vi "Test Post-filter.vi"(8 "error in (no error)":errorcluster, 11 "Lockin.DAQ in":refnum<class "Instrument.DAQ.lvclass">) -> (0 "error out":errorcluster, 3 "Lockin.DAQ out":refnum<class "Instrument.DAQ.lvclass">)   [LabVIEW 2019, in "Instrument.Lockin.lvlib" / "Instrument.DAQ.lvclass"]
uses:
  Instrument.DAQ.lvclass
  DSP/DSP.lvclass
  Typedefs/AO.Channel.Function--Enum.ctl
  Typedefs/AO.Channel--Cluster--Array.ctl
  Typedefs/REF.Channel--Cluster--Array.ctl
  Typedefs/DAQ.Sampling.Sampling--Cluster.ctl
  Typedefs/AO.Channel--Cluster.ctl
  Typedefs/REF.Channel--Cluster.ctl
  Typedefs/AI.Channel--Cluster.ctl
  Typedefs/AI.Channel--Cluster--Array.ctl
panel:
  out "appended array":waveform(dbl)[](array[waveform])
  out "Waveform Graph":waveform(dbl)[](graph)
  in  "AI Channels":T1 {"References" items=["", "1", "2", "3"]; "Channel" min=1}
  in  "REF Channels":T3 {"Roll-Off" min=1; "TC" min=0.0001 format="%#_3p"; "Phase" format="%.3g"; "Frequency" min=0.0001 max=10000.0 format="%.3g"; "Channel" min=1}
  in  "sampling":T5={"Fs"=204789.0, "#s"=15753} {"Fs" format="%#_13g"}
  in  "stop":bool
  in  "AO Channels":T6=[{"Enable?"=FALSE, "Channel"=0, "Amplitude"=0.0, "Offset"=0.0, "Frequency"=0.1, "Phase"=0.0, "Function"=enum."Sine", "Sweeping?"=FALSE, "Limit AC"=FALSE, "Limit DC?"=FALSE}] {"Phase" format="%.2g"; "Frequency" min=0.0001 max=10000.0 format="%.2g"; "Offset" format="%5.2p"; "Amplitude" min=0.0 max=10.0 format="%5.2p"}
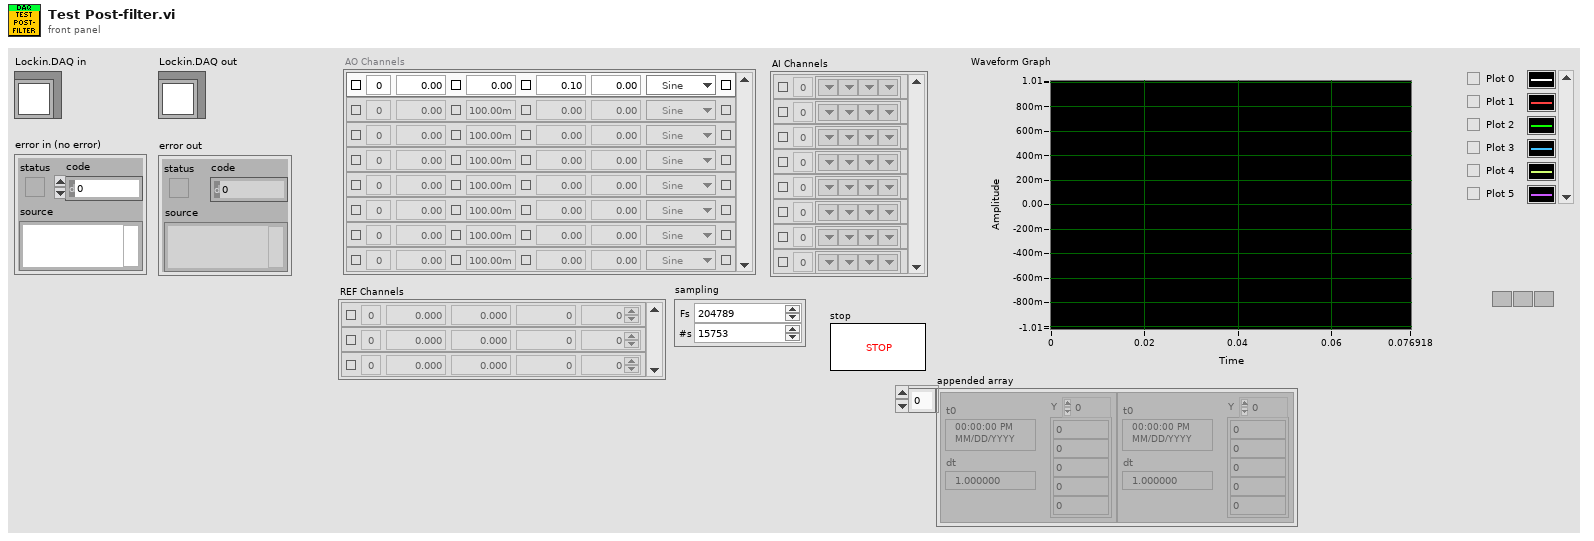
[diagram p1: front panel]
types:
  T1 = typedef "Instrument.Lockin.lvlib/Instrument.DAQ.lvclass/AI.Channel--Cluster--Array.ctl" = T2[]
  T2 = typedef "Instrument.Lockin.lvlib/Instrument.DAQ.lvclass/AI.Channel--Cluster.ctl" = cluster{"Enable?":bool, "Channel":i32, "References":i32[]}
  T3 = typedef "Instrument.Lockin.lvlib/Instrument.DAQ.lvclass/REF.Channel--Cluster--Array.ctl" = T4[]
  T4 = typedef "Instrument.Lockin.lvlib/Instrument.DAQ.lvclass/REF.Channel--Cluster.ctl" = cluster{"Enable?":bool, "Channel":i32, "Frequency":dbl, "Phase":dbl, "TC":dbl, "Roll-Off":i32}
  T5 = typedef "Instrument.Lockin.lvlib/Instrument.DAQ.lvclass/DAQ.Sampling.Sampling--Cluster.ctl" = cluster{"Fs":dbl, "#s":i32}
  T6 = typedef "Instrument.Lockin.lvlib/Instrument.DAQ.lvclass/AO.Channel--Cluster--Array.ctl" = T7[]
  T7 = typedef "Instrument.Lockin.lvlib/Instrument.DAQ.lvclass/AO.Channel--Cluster.ctl" = cluster{"Enable?":bool, "Channel":i32, "Amplitude":dbl, "Offset":dbl, "Frequency":dbl, "Phase":dbl, "Function":T8, "Sweeping?":bool, "Limit AC":bool, "Limit DC?":bool}
  T8 = typedef "Instrument.Lockin.lvlib/Instrument.DAQ.lvclass/AO.Channel.Function--Enum.ctl" = enum16{"Sine", "Triangle", "Square"}
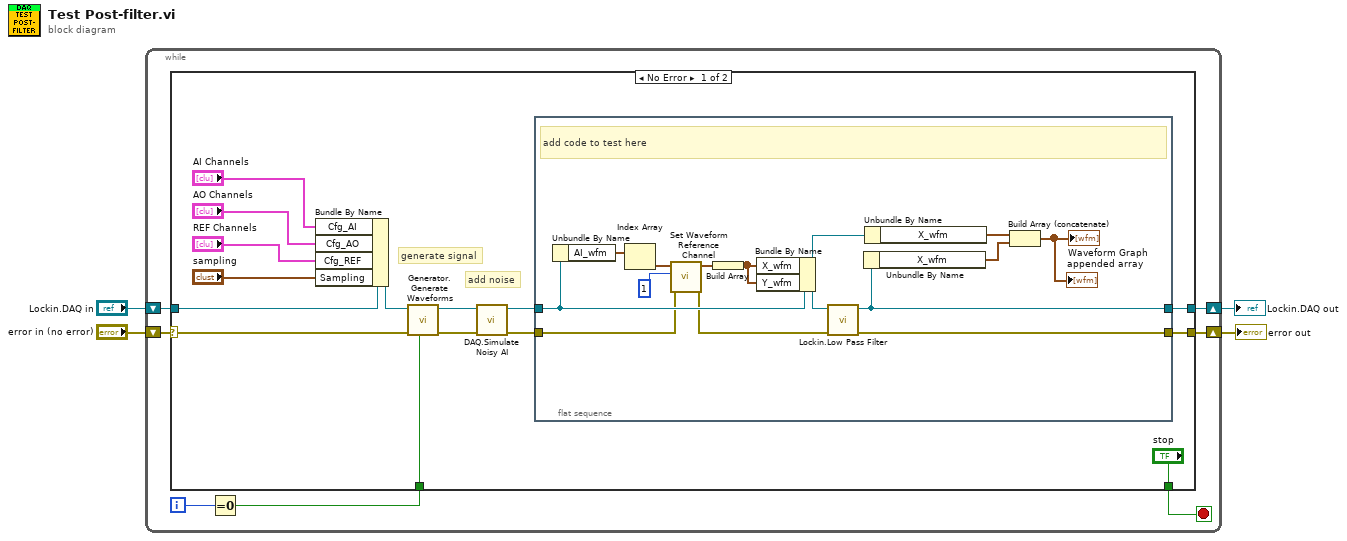
[diagram p0: block diagram]
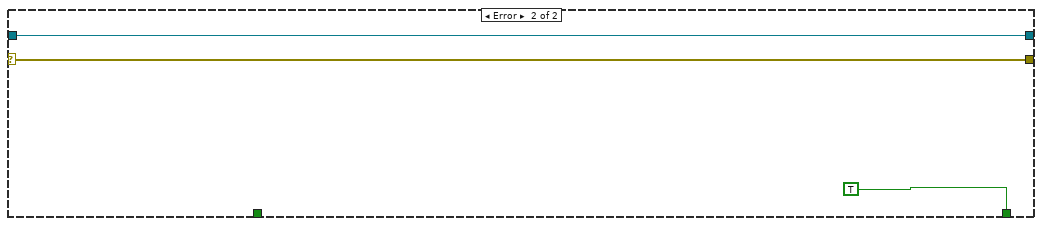
[diagram p2: hidden frame]
diagram:
  n1 = while {
    shift-right: [w10] -> w3
    shift-left: "error in (no error)" -> [w11]
    shift-right: [w8] -> w1
    shift-left: "Lockin.DAQ in" -> [w9]
    i -> [w6]
    stop <- w5 stop-if-true
    n2 = Equal To 0?(x=w6) -> (x = 0?=w7:bool)
    n3 = case shown="No Error" w11 {
      selector: w11 -> [w25 w43]
      tunnel: [w22 w43] -> w10
      tunnel: [w24 w42] -> w8
      tunnel: w9 -> [w15 w42]
      tunnel: w7 -> [w21 _]
      tunnel: ["stop" TRUE ("stop")] -> w5
      frame No Error {
        # "generate signal"
        # "add noise"
        n4 = Bundle By Name(cluster=w15, "Cfg_AI"="AI Channels", "Cfg_AO"="AO Channels", "Cfg_REF"="REF Channels", "Sampling"="sampling") -> (w16:refnum<class "Instrument.DAQ.lvclass">)
        n5 = call "Generator.Generate Waveforms.vi"("Reset Phase?"=w21, "error in (no error)"=w25, "Instrument.DAQ"=w16) -> ("error out"=w26:errorcluster, "Instrument.DAQ"=w12:refnum<class "Instrument.DAQ.lvclass">)  [unwired: 7 in]
        n6 = call "DAQ.Simulate Noisy AI.vi"("error in (no error)"=w26, "Instrument.DAQ in"=w12) -> ("error out"=w23:errorcluster, "Instrument.DAQ out"=w13:refnum<class "Instrument.DAQ.lvclass">)  [unwired: 6 in, 2 out]
        n7 = flat-sequence {
          tunnel: [w35] -> w24
          tunnel: w23 -> [w28]
          tunnel: [w40] -> w22
          tunnel: w13 -> [w39]
          frame #0 {
            # "add code to test here"
            n8 = Unbundle By Name(w39) -> ("AI_wfm"=w33:waveform(dbl)[])
            n9 = Index Array(array=w33) -> (element=w31:waveform(dbl))  [unwired: 1 in]
            n10 = call "Set Waveform Reference Channel.vi"("error in (no error)"=w28, "Reference Ch"=1, "Waveform in"=w31) -> ("error out"=w27:errorcluster, "Waveform out"=w30:waveform(dbl))  [unwired: 7 in]
            n11 = Build Array(w30) -> (w29:waveform(dbl)[])
            n12 = Bundle By Name(cluster=w39, "X_wfm"=w29, "Y_wfm"=w29) -> (w38:refnum<class "Instrument.DAQ.lvclass">)
            n13 = call "Lockin.Low Pass Filter.vi"("error in (no error)"=w27, "Lockin.DAQ"=w38) -> ("error out"=w40:errorcluster, "Lockin.DAQ"=w35:refnum<class "Instrument.DAQ.lvclass">)  [unwired: 8 in]
            n14 = Unbundle By Name(w35) -> ("X_wfm"=w36:waveform(dbl)[])
            n15 = Unbundle By Name(w38) -> ("X_wfm"=w37:waveform(dbl)[])
            n16 = Build Array (concatenate)(w37, w36) -> (→"Waveform Graph" →"appended array":waveform(dbl)[])
          }
        }
      }
      frame Error {
      }
    }
  }
  "error out" <- w3
  "Lockin.DAQ out" <- w1
